vi "Find Library in ProjectItem.vi"(8 "error in (no error)":errorcluster, 10 "Library Name":string="MyClass.lvclass", 11 "ProjectItem in":refnum<vi>) -> (0 "error out":errorcluster, 1 "Found?":bool, 2 "Library out":refnum<vi>, 3 "ProjectItem out":refnum<vi>)   [LabVIEW 2020, in "gRPC Scripting Tools.lvlib"]
uses:
  gRPC Scripting Tools.lvlib
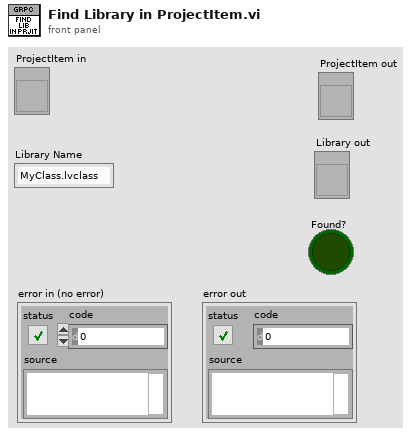
[diagram p1: front panel]
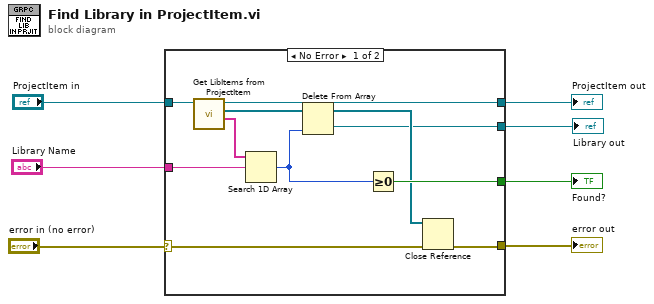
[diagram p0: block diagram]
diagram:
  n1 = case shown="No Error" "error in (no error)" {
    selector: "error in (no error)" -> [w11 w19]
    tunnel: [w10 w19] -> w7
    tunnel: "Library Name" -> [w18 _]
    tunnel: "ProjectItem in" -> [w16 w20]
    tunnel: [w15 w20] -> w3
    tunnel: [w17 _] -> w2
    tunnel: [w8 _] -> w1
    frame No Error {
      n2 = call "Get LibItems from ProjectItem.vi"("ProjectItem in"=w16) -> ("Library Item Names"=w14:string[], "Library Items"=w13:refnum<vi>[], "ProjectItem out"=w15:refnum<vi>)  [unwired: 7 in, 1 out]
      n3 = Search 1D Array(1D array=w14, element=w18) -> (index of element=w12:i32)  [unwired: 1 in]
      n4 = Delete From Array(array=w13, index=w12) -> (deleted portion=w8:refnum<vi>, array with subset deleted=w9:refnum<vi>[])  [unwired: 1 in]
      n5 = Greater Or Equal To 0?(x=w12) -> (x >= 0?=w17:bool)
      n6 = Close Reference(reference=w9, error in (no error)=w11) -> (error out=w10:errorcluster)
    }
    frame Error {
    }
  }
  "error out" <- w7
  "ProjectItem out" <- w3
  "Found?" <- w2
  "Library out" <- w1
